vi "Execute with Process Model.vi"() -> ()   [LabVIEW 2020]
uses:
  SequenceFile/Get Process Model.vi
  SequenceFile/Get Path.vi
  Execution/Set Entry Sequence.vi
  Execution/Set Sequence File.vi
  Execution/Set Process Model.vi
  Execution/Get Result Status.vi
  SequenceFile/SequenceFile.lvclass
  Engine/Engine.lvclass
  Execution/Execution.lvclass
panel:
  in  "Entry Point":string="Single Pass"
  out "Status":string
  in  "Model":T1(tab)
  out "File Model Name":string
  out "Station Model Name":string
  in  "Model Path":path
  in  "SequenceFile Path":path=path "C:/Users/Public/Documents/National Instruments/TestStand 2019 (32-bit)/Examples/Demos/Computer Motherboard Test/LabVIEW/Computer Motherboard Test Sequence.seq"
  # "1."
  # "2."
  # "3."
  # "4."
  # "1. Select the sequence file you'd like to run.\n\n2. Configure the process model you want to run with.\n\n3. If specifying a specific model, select the model file to run with. Otherwise the indicator will update to show the process model that will be used based on the file / station configuration.\n\n4. Enter the name of the entry point to use in the process model. This is usually 'Test UUTs' or 'Single Pass' for models that ship with TestStand."
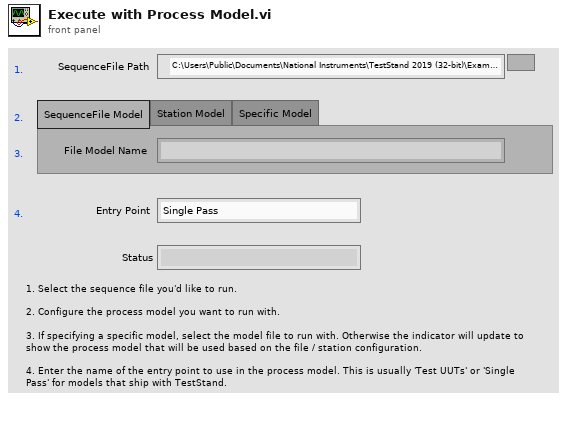
[diagram p1: front panel]
types:
  T1 = enum32{"SequenceFile Model", "Station Model", "Specific Model"}
  T2 = typedef "TSS.lvlib/Engine.lvclass/Session Handle.ctl" = refnum<data-value>
  T3 = typedef "TSS.lvlib/SequenceFile.lvclass/Session Handle.ctl" = refnum<data-value>
  T4 = typedef "TSS.lvlib/Execution.lvclass/Session Handle.ctl" = refnum<data-value>
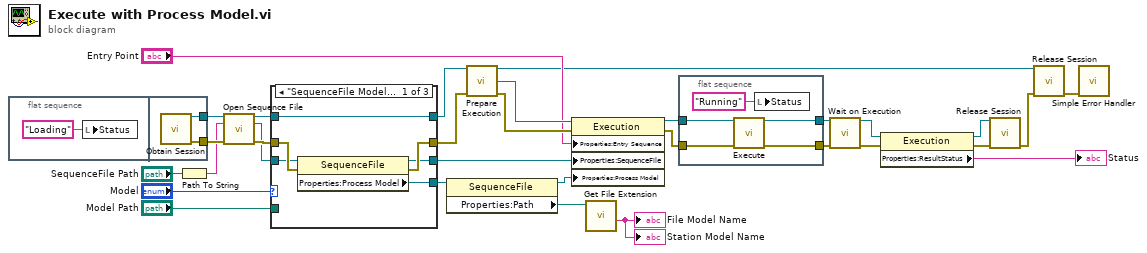
[diagram p0: block diagram]
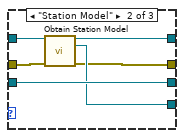
[diagram p2: hidden frame]
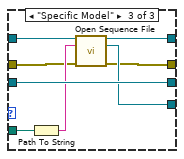
[diagram p3: hidden frame]
diagram:
  n1 = flat-sequence {
    tunnel: [w34] -> w28
    tunnel: [w33] -> w14
    frame #0 {
      n2 = local write "Status"("Loading" ("Status")) -> ()
    }
    frame #1 {
      n3 = call "Obtain Session.vi"() -> ("Session Handle"=w34:T2, "error out"=w33:errorcluster)  [unwired: 14 in]
    }
  }
  n4 = Path To String(path="SequenceFile Path") -> (string=w11:string)
  n5 = call "Open Sequence File.vi"("Session Handle in"=w28, "File Path"=w11, "error in (no error)"=w14) -> ("Session Handle out"=w26:T2, "SequenceFile"=w25:T3, "error out"=w31:errorcluster)  [unwired: 10 in]
  n6 = case shown="\"SequenceFile Model\"" "Model" {
    tunnel: "Model Path" -> [_ _ w53]
    tunnel: w26 -> [w35 w46 w52]
    tunnel: w25 -> [w38 w44 w54]
    tunnel: [w37 w43 w49] -> w24
    tunnel: [w35 w45 w50] -> w21
    tunnel: [w36 w44 w54] -> w7
    tunnel: w31 -> [w40 w42 w48]
    tunnel: [w39 w41 w47] -> w13
    frame "SequenceFile Model" {
      n7 = property class="SequenceFile"(reference=w38, error in=w40) -> (reference out=w36:T3, error out=w39:errorcluster, "Properties:Process Model"=w37:T3)
    }
    frame "Station Model" {
      n8 = call "Obtain Station Model.vi"("Session Handle in"=w46, "error in (no error)"=w42) -> ("Session Handle out"=w45:T2, "Station Model"=w43:T3, "error out"=w41:errorcluster)  [unwired: 11 in]
    }
    frame "Specific Model" {
      n9 = Path To String(path=w53) -> (string=w51:string)
      n10 = call "Open Sequence File.vi"("Session Handle in"=w52, "File Path"=w51, "error in (no error)"=w48) -> ("Session Handle out"=w50:T2, "SequenceFile"=w49:T3, "error out"=w47:errorcluster)  [unwired: 10 in]
    }
  }
  n11 = property class="SequenceFile"(reference=w24) -> (reference out=w19:T3, "Properties:Path"=w23:path)  [unwired: 1 in, 1 out]
  n12 = call "Prepare Execution.vi"("Session Handle in"=w21, "error in (no error)"=w13) -> ("Session Handle out"=w8:T2, "Execution"=w20:T4, "error out"=w12:errorcluster)  [unwired: 11 in]
  n13 = property class="Execution"(reference=w20, error in=w12, "Properties:Entry Sequence"="Entry Point", "Properties:SequenceFile"=w7, "Properties:Process Model"=w19) -> (reference out=w18:T4, error out=w15:errorcluster)
  n14 = call <vilib>:"Get File Extension.vi"("file"=w23) -> ("filename without extension"=→"File Model Name" →"Station Model Name":string)  [unwired: 6 in, 4 out]
  n15 = flat-sequence {
    tunnel: w18 -> [w59]
    tunnel: [w58] -> w17
    tunnel: [w57] -> w16
    tunnel: w15 -> [w56]
    frame #0 {
      n16 = call "Execute.vi"("Session Handle in"=w59, "error in (no error)"=w56) -> ("Session Handle out"=w58:T4, "error out"=w57:errorcluster)  [unwired: 12 in]
      n17 = local write "Status"("Running" ("Status")) -> ()
    }
  }
  n18 = call "Wait on Execution.vi"("Session Handle in"=w17, "error in (no error)"=w16) -> ("Session Handle out"=w6:T4, "error out"=w5:errorcluster)  [unwired: 11 in, 1 out]
  n19 = property class="Execution"(reference=w6, error in=w5) -> (reference out=w3:T4, error out=w4:errorcluster, "Properties:ResultStatus"=→"Status":string)
  n20 = call "Release Session.vi"("Session Handle"=w3, "error in (no error)"=w4) -> ("error out"=w9:errorcluster)  [unwired: 13 in]
  n21 = call "Release Session.vi"("Session Handle"=w8, "error in (no error)"=w9) -> ("error out"=w1:errorcluster)  [unwired: 13 in]
  n22 = call <vilib>:"Simple Error Handler.vi"("error in (no error)"=w1) -> ()  [unwired: 4 in, 5 out]
